vi "Dynamixel Global.vi"() -> ()   [LabVIEW 2022 SP3]
panel:
  in  "Position Backlash":dbl=6.0
  in  "Operating Mode":u8=4
  in  "protocol_version":i32=2
  in  "baud_rate":i32=57600
  in  "Position offset (Deg)":dbl=2.2
  in  "Velocity_profile":u32=10
  in  "Acceleration_profile":u32=20
  in  "Position I Gain Value":u32=1980
  in  "Position P Gain Value":u32=1570
  in  "Position (Deg)":dbl
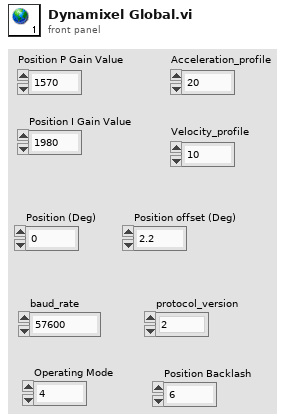
[diagram p1: front panel]
diagram:
